vi "Image UDP Broadcast Initialization VI.vi"(8 "error in (no error)":errorcluster, 10 "Custom XML":string, 11 "Device Item Ref in":T1 format="%.0x") -> (0 "error out":errorcluster, 3 "Device Item Ref out":T1 format="%.0x")   [LabVIEW 2012, in "Image UDP Broadcast Custom Device.lvlib"]
uses:
  Shared/Image UDP Broadcast Custom Device.lvlib
  <vilib>/NI Veristand/Custom Device API/Custom Device Item Ref.ctl
  <vilib>/NI Veristand/Custom Device API/Custom Device Channel.ctl
  <vilib>/NI Veristand/Custom Device API/Custom Device Channel Type.ctl
  Shared/Image UDP Broadcast GUID Lookup.vi
  <vilib>/NI Veristand/Custom Device API/Custom Device API.lvlib
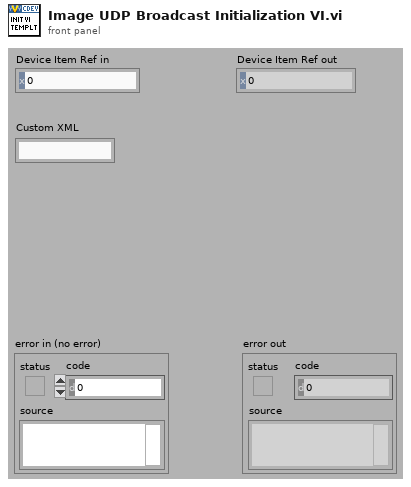
[diagram p1: front panel]
types:
  T1 = typedef "Custom Device API.lvlib/Custom Device Item Ref.ctl" = u64
  T2 = typedef "Custom Device API.lvlib/Custom Device Channel.ctl" = cluster{"Type":T3, "Units":string, "Default Value":dbl, "Faultable":bool, "Scalable":bool}
  T3 = typedef "Custom Device API.lvlib/Custom Device Channel Type.ctl" = enum16{"Input", "Output"}
  T4 = typedef "Image Type" = u32
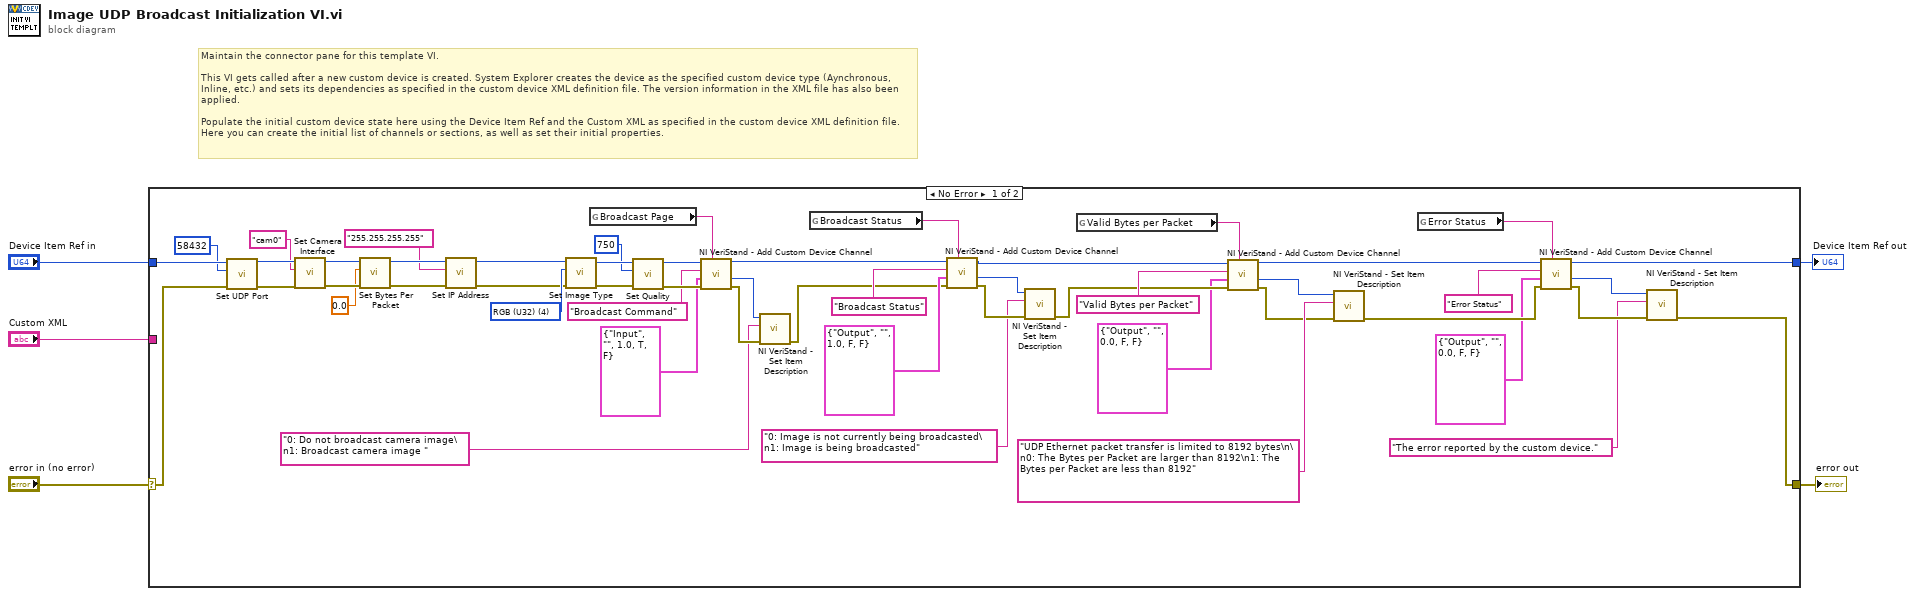
[diagram p0: block diagram]
diagram:
  # "Maintain the connector pane for this template VI.\n\nThis VI gets called after a new custom device is created. System Explorer creates the device as the specified custom device type (Aynchronous, Inline, etc.) and sets its dependencies as specified in the custom device XML definition file. The version information in the XML file has also been applied.\n\nPopulate the initial custom device state here using the Device Item Ref and the Custom XML as specified in the custom device XML definition file. Here you can create the initial list of channels or sections, as well as set their initial properties."
  n1 = case shown="No Error" "error in (no error)" {
    selector: "error in (no error)" -> [w56 w59]
    tunnel: [w14 w59] -> w5
    tunnel: [w15 w58] -> w3
    tunnel: "Device Item Ref in" -> [w57 w58]
    tunnel: "Custom XML" -> [_ _]
    frame No Error {
      w49 = T4 4 items=["Grayscale (U8)", "Grayscale (I16)", "Grayscale (SGL)", "Complex (CSG)", "RGB (U32)", "HSL (U32)", "RGB (U64)", "Grayscale (U16)"] ("Image Type")
      n2 = call "Set UDP Port.vi"("error in (no error)"=w56, "Value"=u16 58432, "Dev Ref in"=w57) -> ("error out"=w54:errorcluster, "Dev Ref out"=w53:T1)  [unwired: 7 in]
      n3 = call "Set Camera Interface.vi"("error in (no error)"=w54, "Value"="cam0", "Dev Ref in"=w53) -> ("error out"=w51:errorcluster, "Dev Ref out"=w50:T1)  [unwired: 7 in]
      n4 = call "Set Bytes Per Packet.vi"("error in (no error)"=w51, "Value"=0.0, "Dev Ref in"=w50) -> ("error out"=w11:errorcluster, "Dev Ref out"=w10:T1)  [unwired: 7 in]
      n5 = call "Set IP Address.vi"("error in (no error)"=w11, "Value"="255.255.255.255", "Dev Ref in"=w10) -> ("error out"=w8:errorcluster, "Dev Ref out"=w9:T1)  [unwired: 7 in]
      n6 = call "Set Image Type.vi"("error in (no error)"=w8, "Value"=w49, "Dev Ref in"=w9) -> ("error out"=w48:errorcluster, "Dev Ref out"=w47:T1)  [unwired: 7 in]
      n7 = global read "Image UDP Broadcast GUID Lookup.vi" "Broadcast Page"() -> (w40:string)
      n8 = call "Set Quality.vi"("error in (no error)"=w48, "Value"=750, "Dev Ref in"=w47) -> ("error out"=w45:errorcluster, "Dev Ref out"=w44:T1)  [unwired: 7 in]
      n9 = call <vilib>:"NI VeriStand - Add Custom Device Channel.vi"("GUID (Default Channel)"=w40, "error in (no error)"=w45, "Channel"=T2 {"Type"=enum."Input", "Units"="", "Default Value"=1.0, "Faultable"=TRUE, "Scalable"=FALSE}, "Channel Name"="Broadcast Command", "Parent Ref in"=w44) -> ("error out"=w37:errorcluster, "Channel Ref"=w36:T1, "Parent Ref out"=w41:T1)  [unwired: 3 in, 1 out]
      n10 = call <vilib>:"NI VeriStand - Set Item Description.vi"("error in (no error)"=w37, "Description"="0: Do not broadcast camera image\n1: Broadcast camera image ", "Item Ref in"=w36) -> ("error out"=w35:errorcluster)  [unwired: 6 in, 2 out]
      n11 = global read "Image UDP Broadcast GUID Lookup.vi" "Broadcast Status"() -> (w33:string)
      n12 = call <vilib>:"NI VeriStand - Add Custom Device Channel.vi"("GUID (Default Channel)"=w33, "error in (no error)"=w35, "Channel"=T2 {"Type"=enum."Output", "Units"="", "Default Value"=1.0, "Faultable"=FALSE, "Scalable"=FALSE}, "Channel Name"="Broadcast Status", "Parent Ref in"=w41) -> ("error out"=w32:errorcluster, "Channel Ref"=w31:T1, "Parent Ref out"=w24:T1)  [unwired: 3 in, 1 out]
      n13 = call <vilib>:"NI VeriStand - Set Item Description.vi"("error in (no error)"=w32, "Description"="0: Image is not currently being broadcasted\n1: Image is being broadcasted", "Item Ref in"=w31) -> ("error out"=w23:errorcluster)  [unwired: 6 in, 2 out]
      n14 = global read "Image UDP Broadcast GUID Lookup.vi" "Valid Bytes per Packet"() -> (w26:string)
      n15 = call <vilib>:"NI VeriStand - Add Custom Device Channel.vi"("GUID (Default Channel)"=w26, "error in (no error)"=w23, "Channel"=T2 {"Type"=enum."Output", "Units"="", "Default Value"=0.0, "Faultable"=FALSE, "Scalable"=FALSE}, "Channel Name"="Valid Bytes per Packet", "Parent Ref in"=w24) -> ("error out"=w27:errorcluster, "Channel Ref"=w28:T1, "Parent Ref out"=w16:T1)  [unwired: 3 in, 1 out]
      n16 = call <vilib>:"NI VeriStand - Set Item Description.vi"("error in (no error)"=w27, "Description"="UDP Ethernet packet transfer is limited to 8192 bytes\n\n0: The Bytes per Packet are larger than 8192\n1: The Bytes per Packet are less than 8192", "Item Ref in"=w28) -> ("error out"=w13:errorcluster)  [unwired: 6 in, 2 out]
      n17 = global read "Image UDP Broadcast GUID Lookup.vi" "Error Status"() -> (w20:string)
      n18 = call <vilib>:"NI VeriStand - Add Custom Device Channel.vi"("GUID (Default Channel)"=w20, "error in (no error)"=w13, "Channel"=T2 {"Type"=enum."Output", "Units"="", "Default Value"=0.0, "Faultable"=FALSE, "Scalable"=FALSE}, "Channel Name"="Error Status", "Parent Ref in"=w16) -> ("error out"=w19:errorcluster, "Channel Ref"=w18:T1, "Parent Ref out"=w15:T1)  [unwired: 3 in, 1 out]
      n19 = call <vilib>:"NI VeriStand - Set Item Description.vi"("error in (no error)"=w19, "Description"="The error reported by the custom device.", "Item Ref in"=w18) -> ("error out"=w14:errorcluster)  [unwired: 6 in, 2 out]
    }
    frame Error {
    }
  }
  "error out" <- w5
  "Device Item Ref out" <- w3
